vi "Analysis.Fail Paredo, Merge All, FP,a nd LP to table_V2.vi"(9 "LP Pareto":string[][](table), 10 "FP Pareto":string[][](table), 11 "All Pareto":string[][](table)) -> (3 "Failure Pareto":string[][](table))   [LabVIEW 2024]
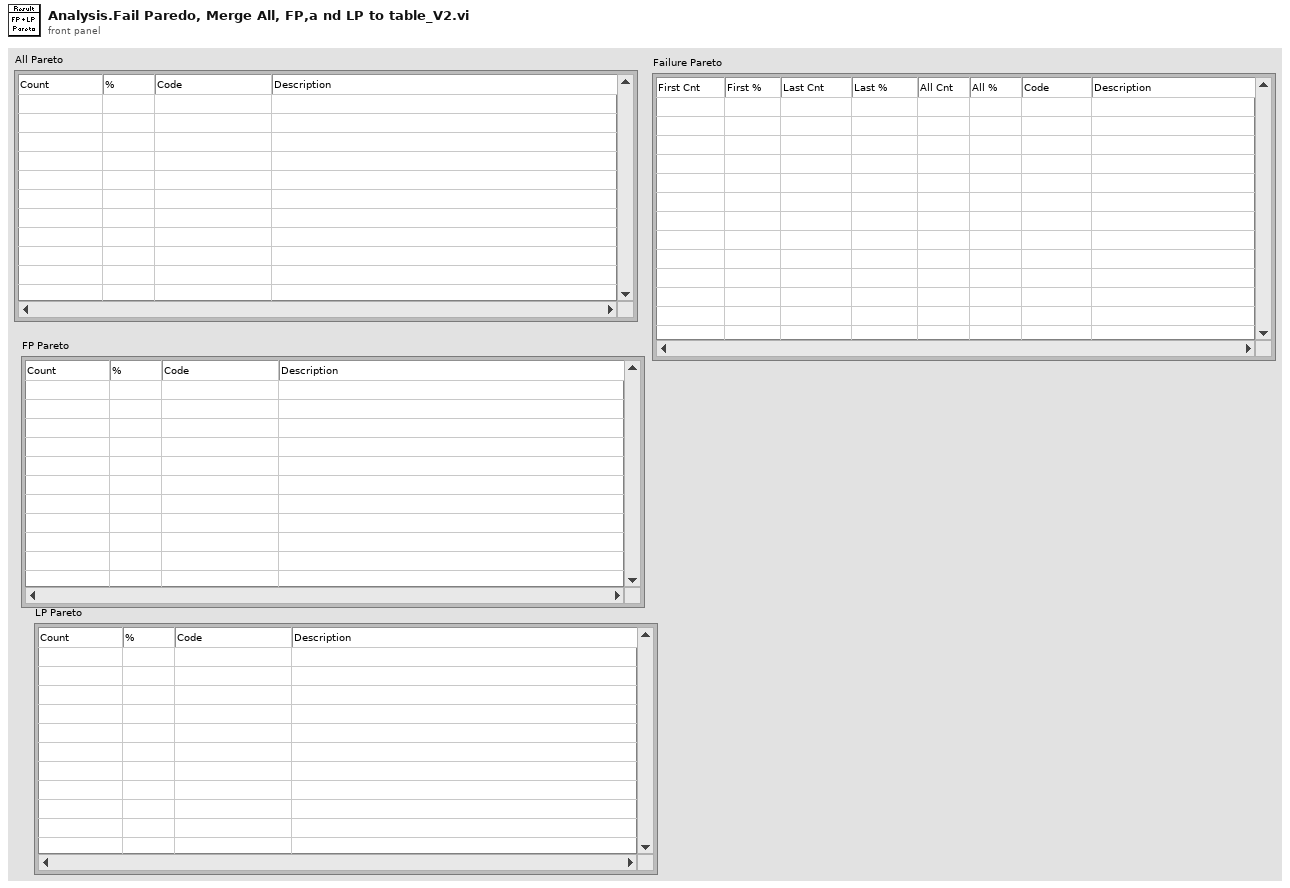
[diagram p1: front panel]
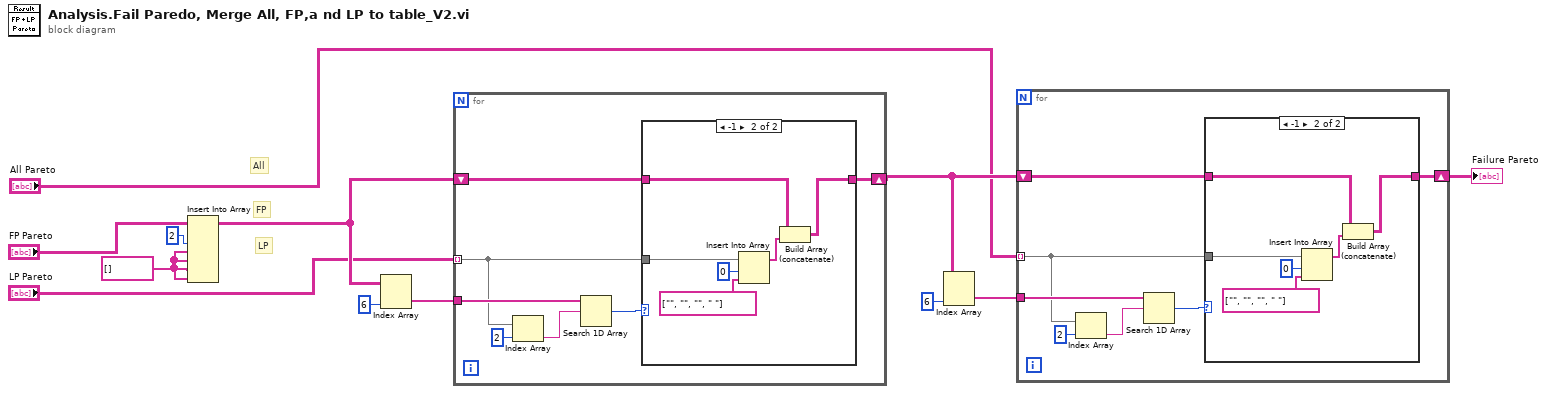
[diagram p0: block diagram]
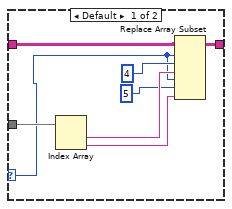
[diagram p2: hidden frame]
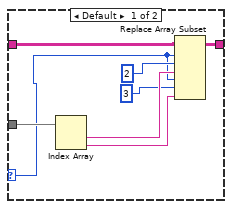
[diagram p3: hidden frame]
diagram:
  w8 = string[] []
  # "LP"
  # "FP"
  # "All"
  n1 = Insert Into Array(array="FP Pareto", index (col)=2 ("index (row)"), new element #1=w8, new element #2=w8, new element #3=w8, new element #4=w8) -> (w12:string[][])  [unwired: 1 in]
  n2 = Index Array(array=w12, index (col)=6 ("index (row)")) -> (element=w10:string[])  [unwired: 1 in]
  n3 = for {
    tunnel: "LP Pareto" -> [w14] mode=indexing
    tunnel: w10 -> [w18]
    shift-right: [w13] -> w4
    shift-left: w12 -> [w16]
    n4 = Index Array(array=w14, index=2) -> (element=w17:string)
    n5 = Search 1D Array(1D array=w18, element=w17) -> (index of element=w15:i32)  [unwired: 1 in]
    n6 = case shown="-1" w15 {
      selector: w15 -> [w22 _]
      tunnel: w16 -> [w25 w33]
      tunnel: w14 -> [w27 w32]
      tunnel: [w26 w28] -> w13
      frame Default {
        n7 = Index Array(array=w27) -> (element #1=w23:string, element #2=w20:string)  [unwired: 2 in]
        n8 = Replace Array Subset(array=w25, new element #1=w23, index (row) #1=w22, index (col) #1=2 ("disabled index (col)"), new element #2=w20, index (row) #2=w22, index (col) #2=3 ("disabled index (col)")) -> (w26:string[][])
      }
      frame -1 {
        n9 = Insert Into Array(array=w32, index=0, new element=string[] ["", "", "", " "]) -> (w29:string[])
        n10 = Build Array (concatenate)(w33, w29) -> (w28:string[][])
      }
    }
  }
  n11 = Index Array(array=w4, index (col)=6 ("index (row)")) -> (element=w7:string[])  [unwired: 1 in]
  n12 = for {
    tunnel: "All Pareto" -> [w35] mode=indexing
    tunnel: w7 -> [w39]
    shift-right: [w34] -> w5
    shift-left: w4 -> [w37]
    n13 = Index Array(array=w35, index=2) -> (element=w38:string)
    n14 = Search 1D Array(1D array=w39, element=w38) -> (index of element=w36:i32)  [unwired: 1 in]
    n15 = case shown="-1" w36 {
      selector: w36 -> [w43 _]
      tunnel: w37 -> [w46 w54]
      tunnel: w35 -> [w48 w53]
      tunnel: [w47 w49] -> w34
      frame Default {
        n16 = Index Array(array=w48) -> (element #1=w44:string, element #2=w41:string)  [unwired: 2 in]
        n17 = Replace Array Subset(array=w46, new element #1=w44, index (row) #1=w43, index (col) #1=4 ("disabled index (col)"), new element #2=w41, index (row) #2=w43, index (col) #2=5 ("disabled index (col)")) -> (w47:string[][])
      }
      frame -1 {
        n18 = Insert Into Array(array=w53, index=0, new element=string[] ["", "", "", " "]) -> (w50:string[])
        n19 = Build Array (concatenate)(w54, w50) -> (w49:string[][])
      }
    }
  }
  "Failure Pareto" <- w5
